vi "Switch Configuration - ab0 exists.vi"(8 "error in (no error)":errorcluster, 9 "Topology Data":T1) -> (0 "error out":errorcluster, 2 "ab0 Exists?":bool)   [LabVIEW 2015, in "DMM-SWITCH-ScanList System Explorer.lvlib"]
doc: "Reads the Switch Top File for the selected Topology and verifies if ab0 exists."
uses:
  DMM-SWITCH-ScanList System Explorer.lvlib
  Configuration Controls/Topology Data.ctl
  <vilib>/Utility/sysdir.llb/System Directory Type.ctl
  Shared/Constants.vi
  Shared/DMM-SWITCH-ScanList Shared.lvlib
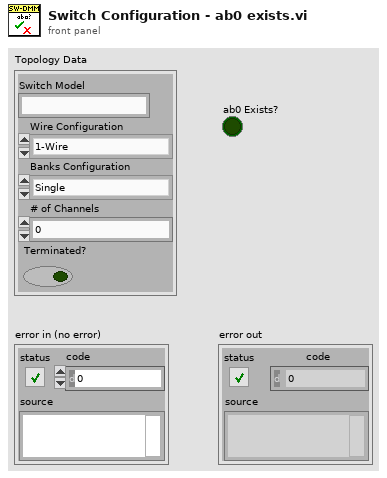
[diagram p1: front panel]
types:
  T1 = typedef "DMM-SWITCH-ScanList System Explorer.lvlib/Topology Data.ctl" = cluster{"Switch Model":string, "Wire Configuration":enum16{"1-Wire", "2-Wire", "4-Wire"}, "Banks Configuration":enum16{"Single", "Dual", "Quad", "Octal", "Sixteen"}, "# of Channels":u32, "Terminated?":bool}
  T2 = typedef "System Directory Type.ctl" = i32
  T3 = enum16{"Single", "Dual", "Quad", "Octal", "Sixteen"}
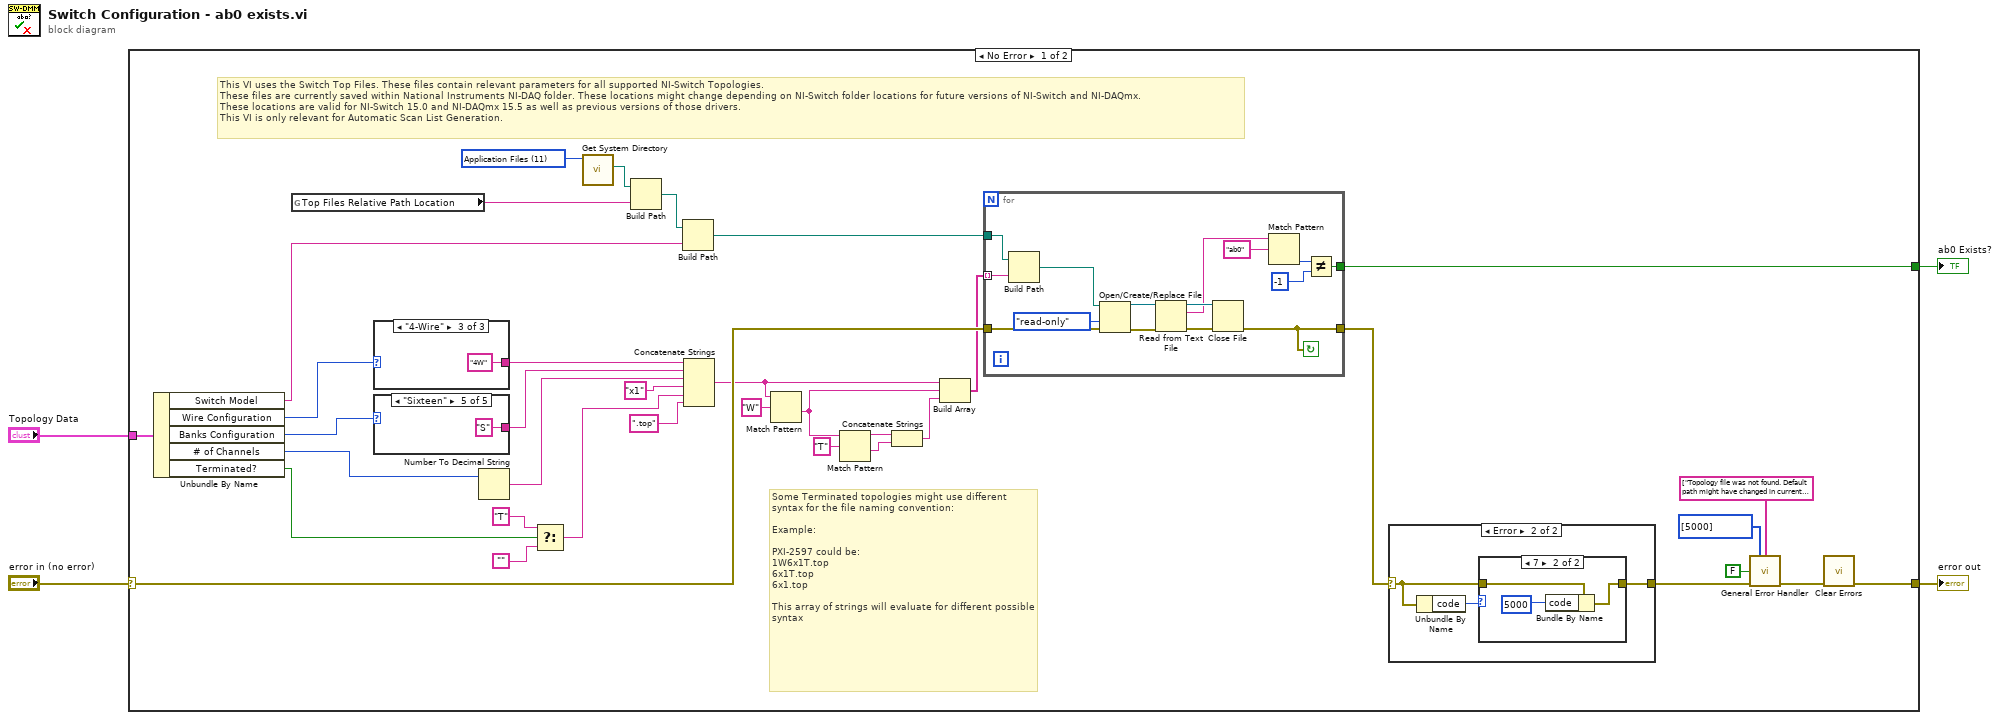
[diagram p0: block diagram]
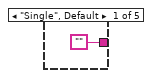
[diagram p4: hidden frame]
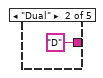
[diagram p5: hidden frame]
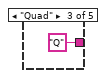
[diagram p6: hidden frame]
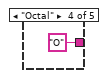
[diagram p7: hidden frame]
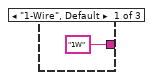
[diagram p8: hidden frame]
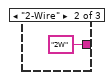
[diagram p9: hidden frame]
diagram:
  n1 = case shown="No Error" "error in (no error)" {
    selector: "error in (no error)" -> [w29 w72]
    tunnel: "Topology Data" -> [w37 _]
    tunnel: [w30 _] -> w3
    tunnel: [w5 w72] -> w1
    frame No Error {
      w40 = T2 11 items=["User Home"=0, "User Desktop"=1, "User Documents"=2, "User Application Data"=3, "User Preferences"=4, "User Temporary"=5, "Public Documents"=6, "Public Application Data"=7, "Public Preferences"=8, "Public Cache"=13, "System Core Libraries"=9, "System Installed Libraries"=10, "Application Files"=11, "Boot Volume Root"=12] ("system directory type")
      # "Some Terminated topologies might use different syntax for the file naming convention:\n \nExample:\n\nPXI-2597 could be:\n1W6x1T.top\n6x1T.top\n6x1.top\n\nThis array of strings will evaluate for different possible syntax"
      # "This VI uses the Switch Top Files. These files contain relevant parameters for all supported NI-Switch Topologies. \nThese files are currently saved within National Instruments NI-DAQ folder. These locations might change depending on NI-Switch folder locations for future versions of NI-Switch and NI-DAQmx.\nThese locations are valid for NI-Switch 15.0 and NI-DAQmx 15.5 as well as previous versions of those drivers.\nThis VI is only relevant for Automatic Scan List Generation."
      n2 = Unbundle By Name(w37) -> ("Switch Model"=w28:string, "Wire Configuration"=w36:enum16{"1-Wire", "2-Wire", "4-Wire"}, "Banks Configuration"=w35:T3, "# of Channels"=w34:u32, "Terminated?"=w27:bool)
      n3 = global read "Constants.vi" "Top Files Relative Path Location"() -> (w11:string)
      n4 = case shown="\"4-Wire\"" w36 {
        tunnel: ["1W" "2W" "4W"] -> w33
        frame "1-Wire", Default {
        }
        frame "2-Wire" {
        }
        frame "4-Wire" {
        }
      }
      n5 = case shown="\"Sixteen\"" w35 {
        tunnel: ["" "D" "Q" "O" "S"] -> w32
        frame "Single", Default {
        }
        frame "Dual" {
        }
        frame "Quad" {
        }
        frame "Octal" {
        }
        frame "Sixteen" {
        }
      }
      n6 = Number To Decimal String(number=w34) -> (decimal integer string=w31:string)  [unwired: 1 in]
      n7 = Select(t="T", s=w27, f="") -> (s? t:f=w23:string)
      n8 = call <vilib>:"Get System Directory.vi"("system directory type"=w40) -> ("system directory"=w39:path)  [unwired: 10 in]
      n9 = Build Path(base path=w39, name or relative path=w11) -> (appended path=w38:path)
      n10 = Build Path(base path=w38, name or relative path=w28) -> (appended path=w21:path)
      n11 = Concatenate Strings(w33, w32, w31, "x1" ("string"), w23, ".top" ("string")) -> (w19:string)
      n12 = Match Pattern(string=w19, regular expression="W") -> (after substring=w18:string)  [unwired: 1 in, 3 out]
      n13 = Match Pattern(string=w18, regular expression="T") -> (before substring=w16:string, after substring=w15:string)  [unwired: 1 in, 2 out]
      n14 = Concatenate Strings(w16, w15) -> (w14:string)
      n15 = Build Array(w19, w18, w14) -> (w13:string[])
      n16 = for {
        tunnel: [w63] -> w30
        tunnel: w21 -> [w61]
        tunnel: w13 -> [w60] mode=indexing
        tunnel: w29 -> [w62]
        tunnel: [w49] -> w12
        stop <- w49 continue-if-true
        n17 = Build Path(base path=w61, name or relative path=w60) -> (appended path=w59:path)
        n18 = Open/Create/Replace File(file path (use dialog)=w59, error in=w62, access (0:read/write)=enum16{"read/write", "read-only", "write-only"}."read-only") -> (refnum out=w56:refnum<file>, error out=w57:errorcluster)  [unwired: 3 in, 1 out]
        n19 = Read from Text File(file (use dialog)=w56, error in=w57) -> (refnum out=w54:refnum<file>, text=w53:string, error out=w55:errorcluster)  [unwired: 2 in, 1 out]
        n20 = Close File(refnum=w54, error in=w55) -> (error out=w49:errorcluster)  [unwired: 1 out]
        n21 = Match Pattern(string=w53, regular expression="ab0") -> (offset past match=w51:i32)  [unwired: 1 in, 3 out]
        n22 = Not Equal?(x=w51, y=-1) -> (x != y?=w63:bool)
      }
      n23 = case shown="Error" w12 {
        selector: w12 -> [w41 w43]
        tunnel: [w41 w42] -> w7
        frame No Error {
        }
        frame Error {
          n24 = Unbundle By Name(w43) -> ("code"=w44:i32)
          n25 = case shown="7" w44 {
            tunnel: w43 -> [w45 w48]
            tunnel: [w45 w46] -> w42
            frame 0, Default {
            }
            frame 7 {
              n26 = Bundle By Name(cluster=w48, "code"=5000) -> (w46:errorcluster)
            }
          }
        }
      }
      n27 = call <vilib>:"General Error Handler.vi"("[user-defined codes]"=i32[] [5000], "[user-defined descriptions]"=string[] ["Topology file was not found. Default path might have changed in current driver version. Try generating the Scan List Manually using NI-Switch scan list syntax"], "search ni.com link visible?(T)"=FALSE, "error in (no error)"=w7) -> ("error out"=w6:errorcluster)  [unwired: 7 in, 4 out]
      n28 = call <vilib>:"Clear Errors.vi"("error in (no error)"=w6) -> ("error out"=w5:errorcluster)  [unwired: 1 in, 5 out]
    }
    frame Error {
    }
  }
  "ab0 Exists?" <- w3
  "error out" <- w1
